vi "Set Impedance Compensation.vi"(8 "error in (no error)":errorcluster, 10 "Impedance Compensation (0: None)":u32(ring) items=["None", "2 - Wire", "4 - Wire "], 11 "VISA resource name":refnum<visa-resource-name>) -> (0 "error out":errorcluster, 3 "VISA resource name out":refnum<visa-resource-name>)   [LabVIEW 2014, in "Fluke 5XXX Series Multicalibrators.lvlib"]
doc: "This VI activates or deactivates 2-wire or 4-wire impedance compensation. \n\nFour-wire and two-wire connections refer to methods of connecting the calibrator to the UUT to cancel out test lead resistance to assure the highest precision of the calibration output. The external sensing capability of the four-wire and two-wire compensated connections provide increased precision for resistance values below 110 kOhms and capacitance values 110 nF and above.\n\nNote:\n\nThe following 55xxA and 57xxA resistance modes are equivalent:\n\n55xxA 57xxA\nCOMP Off 2 wire Comp OFF, EX SNS off (disabled)\nCOMP 2 wire 2 wire Comp ON, EX SNS on (enabled)\nCOMP 4 wire 2 wire Comp OFF, EX SNS on (enabled)"
uses:
  Fluke 5XXX Series Multicalibrators.lvlib
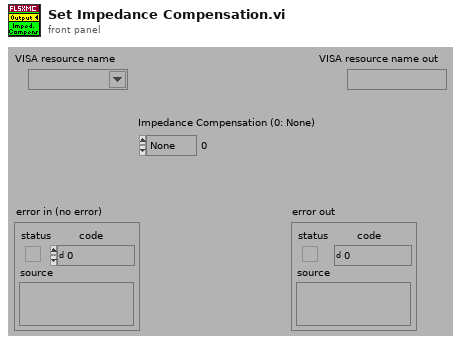
[diagram p1: front panel]
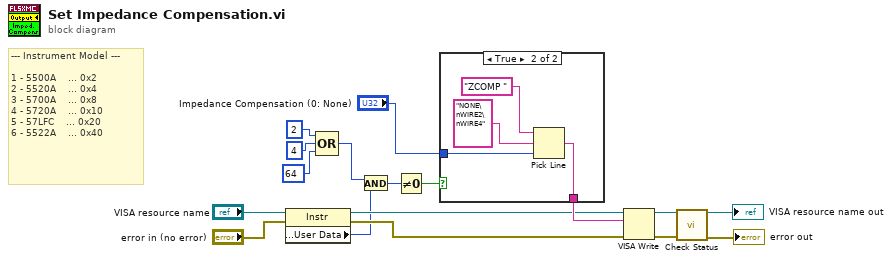
[diagram p0: block diagram]
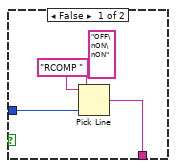
[diagram p2: hidden frame]
diagram:
  # "--- Instrument Model ---\n\n1 - 5500A    ... 0x2\n2 - 5520A    ... 0x4\n3 - 5700A    ... 0x8\n4 - 5720A    ... 0x10\n5 - 57LFC    ... 0x20\n6 - 5522A    ... 0x40"
  n1 = property class="Instr"(reference="VISA resource name", error in="error in (no error)") -> (reference out=w8:refnum<visa-resource-name>, error out=w6:errorcluster, "General Settings:User Data"=w5:u32)
  n2 = Compound Arithmetic op=OR(u32 2 ("Numeric"), u32 4 ("Numeric"), 64 ("Numeric")) -> (w4:u32)
  n3 = And(x=w4, y=w5) -> (x .and. y?=w3:u32)
  n4 = Not Equal To 0?(x=w3) -> (x != 0?=w2:bool)
  n5 = case shown="True" w2 {
    tunnel: [w19 w23] -> w15
    tunnel: "Impedance Compensation (0: None)" -> [w18 w22]
    frame False {
      n6 = Pick Line(string ("")="RCOMP " ("Reset Command"), multi-line string="OFF\nON\nON", line index=w18) -> (output string=w19:string)
    }
    frame True {
      n7 = Pick Line(string ("")="ZCOMP ", multi-line string="NONE\nWIRE2\nWIRE4", line index=w22) -> (output string=w23:string)
    }
  }
  n8 = VISA Write(VISA resource name=w8, write buffer=w15, error in (no error)=w6) -> (VISA resource name out=w17:refnum<visa-resource-name>, error out=w16:errorcluster)  [unwired: 1 out]
  n9 = call "Check Status.vi"("VISA resource name"=w17, "error in (no error)"=w16) -> ("VISA resource name out"=→"VISA resource name out":refnum<visa-resource-name>, "error out"=→"error out":errorcluster)  [unwired: 12 in]
